vi "SpkFilterConnect.vi"(7 "LVWSR":refnum<class "Web Request.lvclass">, 11 "conn":u8) -> ()   [LabVIEW 2014]
uses:
  <vilib>/wsapi/Web Request.lvclass
  Controller/Controller.lvclass
  reusable/Session APIs/CVT/CVT.lvclass
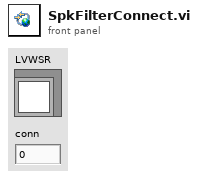
[diagram p1: front panel]
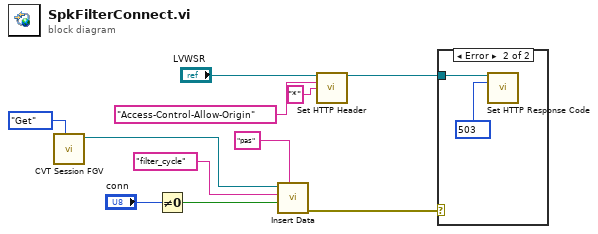
[diagram p0: block diagram]
diagram:
  n1 = call "CVT Session FGV.vi"("State"=enum16{"Init", "Get"}."Get") -> ("CVT Session Out"=w5:refnum<data-value>)  [unwired: 10 in]
  n2 = Not Equal To 0?(x="conn") -> (x != 0?=w2:bool)
  n3 = call "Insert Data.vi"("Group"="pas", "Data"=w2, "tag"="filter_cycle", "CVT Session In"=w5) -> ("error out"=w1:errorcluster)  [unwired: 6 in, 1 out]
  n4 = call <vilib>:"Set HTTP Header.vi"("LabVIEW Web Service Request"="LVWSR", "header"="Access-Control-Allow-Origin", "header value"="*") -> ("LabVIEW Web Service Request out"=w8:refnum<class "Web Request.lvclass">)  [unwired: 11 in, 1 out]
  n5 = case shown="Error" w1 {
    tunnel: w8 -> [_ w12]
    frame No Error {
    }
    frame Error {
      w13 = 503 items=["100"=100, "101"=101, "200"=200, "201"=201, "202"=202, "203"=203, "204"=204, "205"=205, "206"=206, "300"=300, "301"=301, "302"=302, "303"=303, "304"=304, "305"=305, "306"=306, "307"=307, "400"=400, "401"=401, "402"=402, "403"=403, "404"=404, "405"=405, "406"=406, "407"=407, "408"=408, "409"=409, "410"=410, "411"=411, "412"=412, "413"=413, "414"=414, "415"=415, "416"=416, "417"=417, "500"=500, "501"=501, "502"=502, "503"=503, "504"=504, "505"=505] ("response code (200)")
      n6 = call <vilib>:"Set HTTP Response Code.vi"("LabVIEW Web Service Request"=w12, "response code (200)"=w13) -> ()  [unwired: 12 in, 2 out]
    }
  }
